vi "Get_Preview_Cache.vi"(8 "error in (no error)":errorcluster, 11 "AB_Build in":refnum<class "AB_Build.lvclass">) -> (0 "error out":errorcluster, 1 "GeneratedFiles":path[](array[path]), 3 "AB_Build out":refnum<class "AB_Build.lvclass">, 5 "OutputDirectory":path)   [LabVIEW 2020, in "AB_Build.lvclass"]
uses:
  <vilib>/AppBuilder/AB_Classes/Build/AB_Build.lvclass
  <vilib>/AppBuilder/AB_Classes/Build/AB_Build.lvclass/AB_Build.ctl
  <vilib>/AppBuilder/AB_Classes/PreviewCache/PreviewCache.lvclass
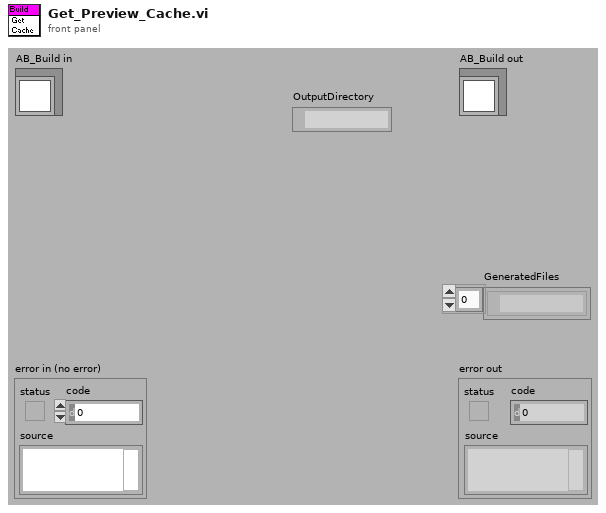
[diagram p1: front panel]
types:
  T1 = typedef "PreviewCache.ctl" = cluster{"build preview data":T2, "project symbol checksum":string, "target symbol checksum":string, "My Computer checksum":string}
  T2 = typedef "build preview data.ctl" = cluster{"generated files":path[], "output directory":path, "buildVersion":cluster{"major":u16, "minor":u16, "patch":u16, "build":u16}}
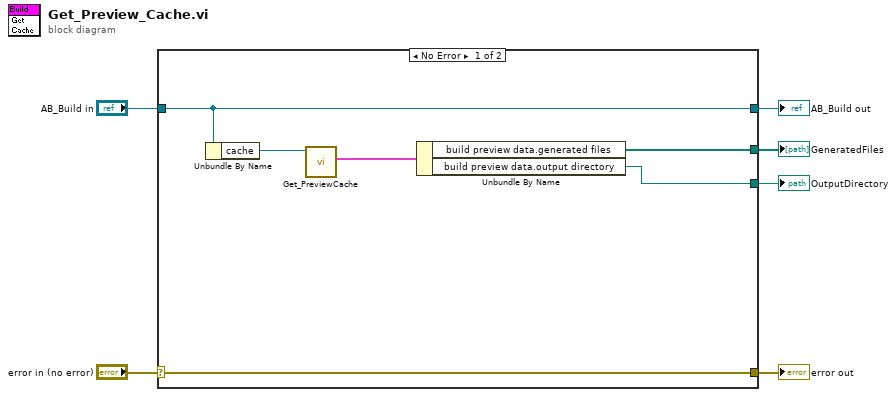
[diagram p0: block diagram]
diagram:
  n1 = case shown="No Error" "error in (no error)" {
    selector: "error in (no error)" -> [w12 w14]
    tunnel: [w12 w14] -> w5
    tunnel: [w11 w13] -> w3
    tunnel: "AB_Build in" -> [w11 w13]
    tunnel: [w8 _] -> w2
    tunnel: [w7 _] -> w1
    frame No Error {
      n2 = Unbundle By Name(w11) -> ("cache"=w10:refnum<class "PreviewCache.lvclass">)
      n3 = call <vilib>:"Get_PreviewCache.vi"("PreviewCache in"=w10) -> ("data"=w9:T1)  [unwired: 8 in, 2 out]
      n4 = Unbundle By Name(w9) -> ("build preview data.generated files"=w8:path[], "build preview data.output directory"=w7:path)
    }
    frame Error {
    }
  }
  "error out" <- w5
  "AB_Build out" <- w3
  "OutputDirectory" <- w1
  "GeneratedFiles" <- w2
